vi "GetApprovedList.vi"(8 "error in (no error)":errorcluster, 11 "ApprovedDeps":T2[](array[typedef])) -> (0 "error out":errorcluster, 3 "Confirmed Deps List":T1[](array[typedef]))   [LabVIEW 2019, in "Hawkeye.lvlib"]
uses:
  Hawkeye.lvlib
  Typedefs/ApprovedDeps.ctl
  Typedefs/ConfirmDeps.ctl
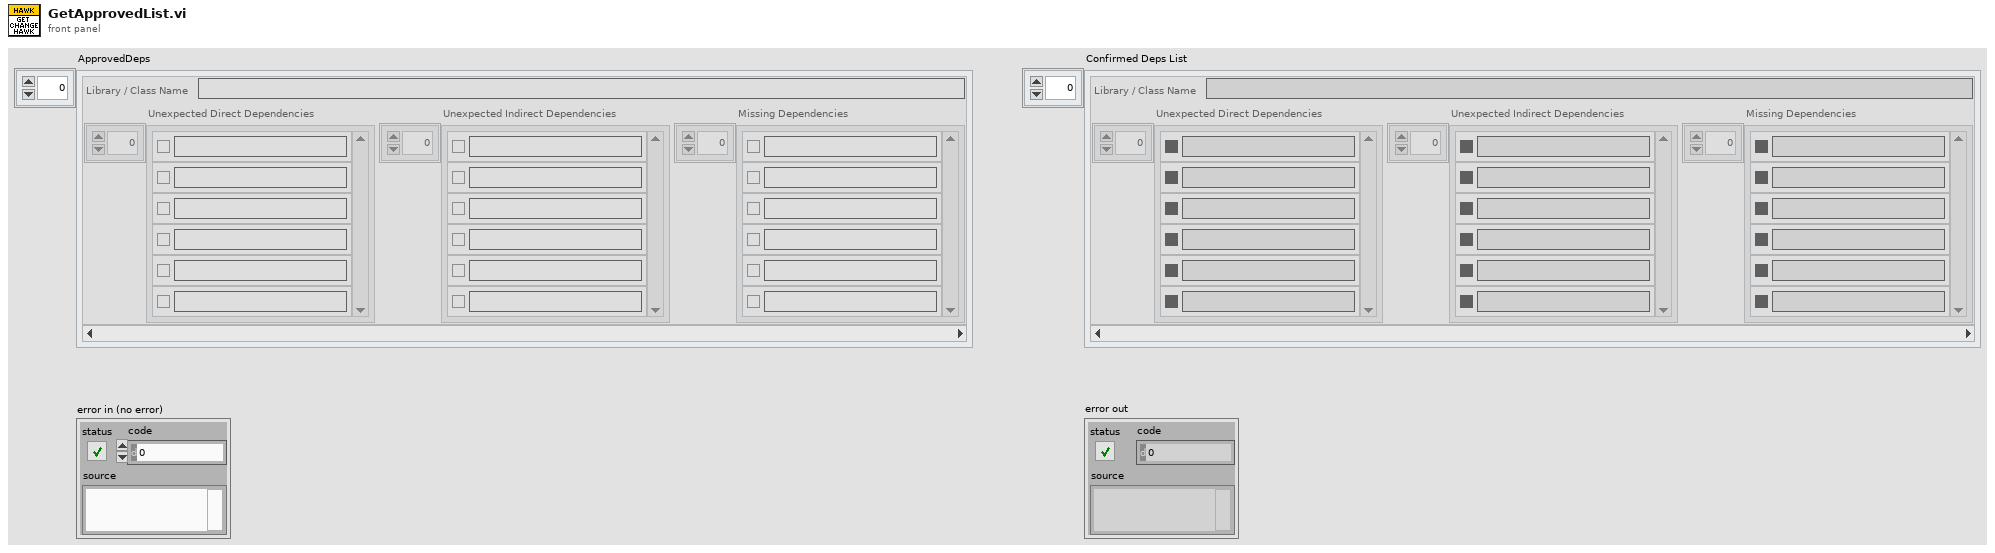
[diagram p1: front panel]
types:
  T1 = typedef "Hawkeye.lvlib/ConfirmDeps.ctl" = cluster{"Library / Class Name":string, "Unexpected Direct Dependencies":cluster{"Confirm Status":enum8{"False", "True", "Mixed"}, "Library / Class Name":string}[], "Unexpected Indirect Dependencies":cluster{"Confirm Status":enum8{"False", "True", "Mixed"}, "Library / Class Name":string}[], "Missing Dependencies":cluster{"Confirm Status":enum8{"False", "True", "Mixed"}, "Library / Class Name":string}[]}
  T2 = typedef "Hawkeye.lvlib/ApprovedDeps.ctl" = cluster{"Library / Class Name":string, "Unexpected Direct Dependencies":cluster{"Approved":bool, "Library / Class Name":string}[], "Unexpected Indirect Dependencies":cluster{"Approved":bool, "Library / Class Name":string}[], "Missing Dependencies":cluster{"Approved":bool, "Library / Class Name":string}[]}
  T3 = cluster{"Confirm Status":enum8{"False", "True", "Mixed"}, "Library / Class Name":string}
  T4 = cluster{"Approved":bool, "Library / Class Name":string}[]
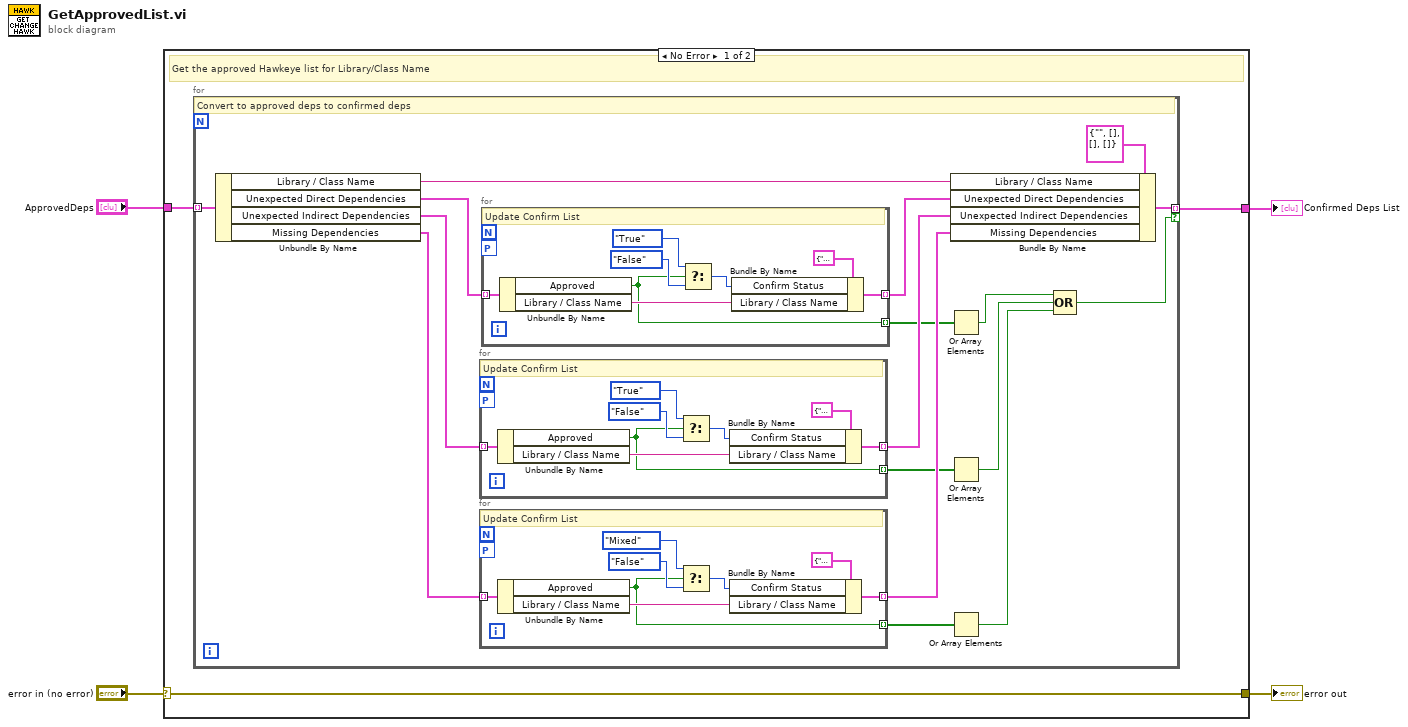
[diagram p0: block diagram]
diagram:
  n1 = case shown="No Error" "error in (no error)" {
    selector: "error in (no error)" -> [w6 w49]
    tunnel: [w6 w49] -> w3
    tunnel: "ApprovedDeps" -> [w7 _]
    tunnel: [w5 _] -> w1
    frame No Error {
      # "Get the approved Hawkeye list for Library/Class Name"
      n2 = for {
        tunnel: w7 -> [w24] mode=indexing
        tunnel: [w18] -> w5 mode=indexing if=w14
        # "Convert to approved deps to confirmed deps"
        n3 = Unbundle By Name(w24) -> ("Library / Class Name"=w22:string, "Unexpected Direct Dependencies"=w21:T4, "Unexpected Indirect Dependencies"=w20:T4, "Missing Dependencies"=w19:T4)
        n4 = for {
          tunnel: w20 -> [w39] mode=indexing
          tunnel: [w34] -> w16 mode=indexing
          workers-P: _ -> [_]
          tunnel: [w33] -> w10 mode=indexing
          # "Update Confirm List"
          n5 = Unbundle By Name(w39) -> ("Approved"=w33:bool, "Library / Class Name"=w38:string)
          n6 = Select(t=enum8{"False", "True", "Mixed"}."True" ("Confirm Status"), s=w33, f=enum8{"False", "True", "Mixed"}."False" ("Confirm Status")) -> (s? t:f=w36:enum8{"False", "True", "Mixed"})
          n7 = Bundle By Name(cluster=T3 {"Confirm Status"=enum."False", "Library / Class Name"=""} ("Unexpected Direct Dependencies"), "Confirm Status"=w36, "Library / Class Name"=w38) -> (w34:T3)
        }
        n8 = for {
          tunnel: w19 -> [w31] mode=indexing
          tunnel: [w26] -> w17 mode=indexing
          workers-P: _ -> [_]
          tunnel: [w25] -> w11 mode=indexing
          # "Update Confirm List"
          n9 = Unbundle By Name(w31) -> ("Approved"=w25:bool, "Library / Class Name"=w30:string)
          n10 = Select(t=enum8{"False", "True", "Mixed"}."Mixed" ("Confirm Status"), s=w25, f=enum8{"False", "True", "Mixed"}."False" ("Confirm Status")) -> (s? t:f=w28:enum8{"False", "True", "Mixed"})
          n11 = Bundle By Name(cluster=T3 {"Confirm Status"=enum."False", "Library / Class Name"=""} ("Unexpected Direct Dependencies"), "Confirm Status"=w28, "Library / Class Name"=w30) -> (w26:T3)
        }
        n12 = for {
          tunnel: w21 -> [w47] mode=indexing
          tunnel: [w42] -> w13 mode=indexing
          workers-P: _ -> [_]
          tunnel: [w41] -> w12 mode=indexing
          # "Update Confirm List"
          n13 = Unbundle By Name(w47) -> ("Approved"=w41:bool, "Library / Class Name"=w46:string)
          n14 = Select(t=enum8{"False", "True", "Mixed"}."True" ("Confirm Status"), s=w41, f=enum8{"False", "True", "Mixed"}."False" ("Confirm Status")) -> (s? t:f=w44:enum8{"False", "True", "Mixed"})
          n15 = Bundle By Name(cluster=T3 {"Confirm Status"=enum."False", "Library / Class Name"=""} ("Unexpected Direct Dependencies"), "Confirm Status"=w44, "Library / Class Name"=w46) -> (w42:T3)
        }
        n16 = Bundle By Name(cluster=T1 {"Library / Class Name"="", "Unexpected Direct Dependencies"=[], "Unexpected Indirect Dependencies"=[], "Missing Dependencies"=[]} ("Confirmed Deps List"), "Library / Class Name"=w22, "Unexpected Direct Dependencies"=w13, "Unexpected Indirect Dependencies"=w16, "Missing Dependencies"=w17) -> (w18:T1)
        n17 = Or Array Elements(Boolean array=w12) -> (logical OR=w15:bool)
        n18 = Or Array Elements(Boolean array=w10) -> (logical OR=w9:bool)
        n19 = Or Array Elements(Boolean array=w11) -> (logical OR=w8:bool)
        n20 = Compound Arithmetic op=OR(w15, w9, w8) -> (w14:bool)
      }
    }
    frame Error {
    }
  }
  "error out" <- w3
  "Confirmed Deps List" <- w1
